vi "fullSERVER - SegnNotDAQ.vi"() -> ()   [LabVIEW 2023]
uses:
  <vilib>/Waveform/WDTFileIO.llb/Read Waveform from File.vi
panel:
  in  "file path (dialog if empty)":path
  out "SIGNAL":waveform(dbl)(graph)
  out "# POINTS":dbl
  out "OBSERVATION TIME":dbl
  out "SAMPLING FREQUENCY":dbl
  in  "PORT":u16
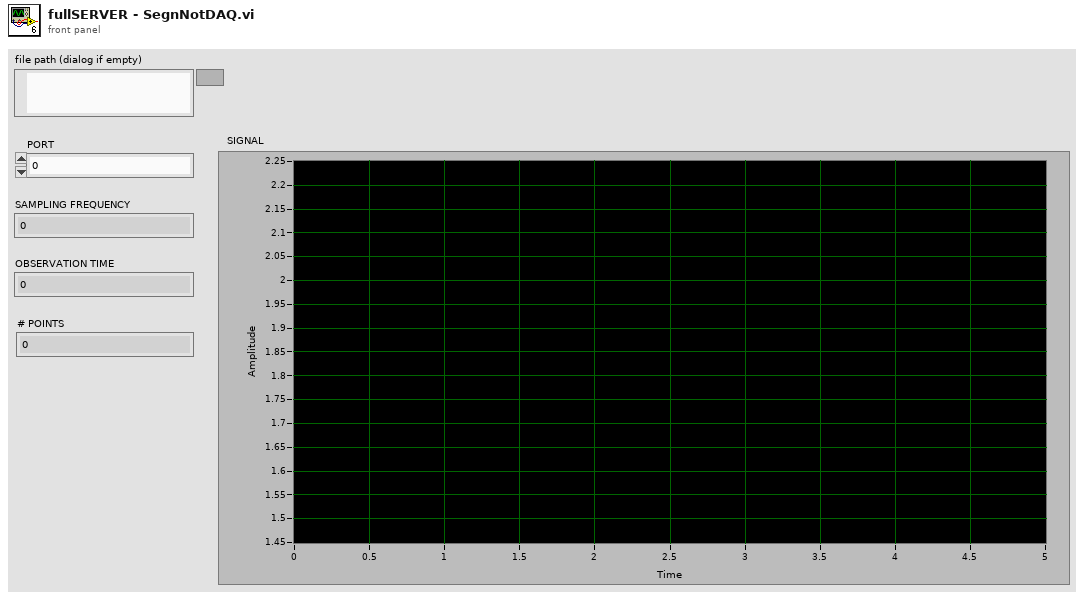
[diagram p1: front panel]
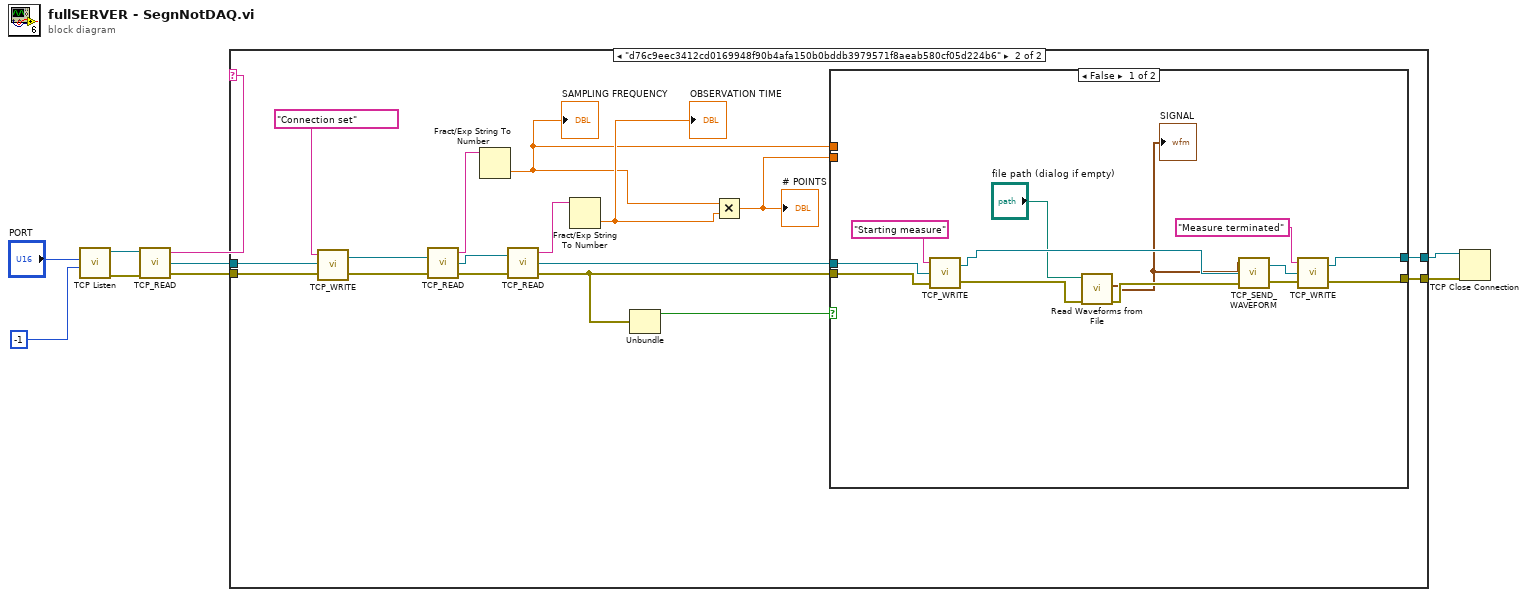
[diagram p0: block diagram]
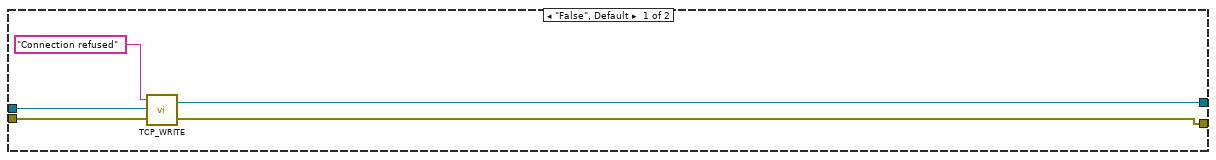
[diagram p2: hidden frame]
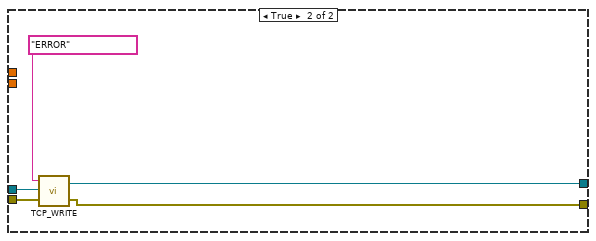
[diagram p3: hidden frame]
diagram:
  n1 = call <vilib>:"TCP Listen.vi"("timeout ms (wait forever: -1)"=-1, "port"="PORT") -> ("error out"=w6:errorcluster, "connection ID"=w7:refnum<k5>)  [unwired: 5 in, 3 out]
  n2 = call "TCP_READ.vi"("connection ID"=w7, "error in (no error)"=w6) -> ("data"=w5:string, "connection ID out"=w4:refnum<k5>, "error out"=w3:errorcluster)
  n3 = case shown="\"d76c9eec3412cd0169948f90b4afa150b0bddb3979571f8aeab580cf05d224b6\"" w5 {
    tunnel: w4 -> [w13 w30]
    tunnel: w3 -> [w14 w31]
    tunnel: [w12 w17] -> w2
    tunnel: [w11 w18] -> w1
    frame "False", Default {
      n4 = call "TCP_WRITE.vi"("error in (no error)"=w14, "connection ID"=w13, "data"="Connection refused") -> ("error out"=w11:errorcluster, "connection ID out"=w12:refnum<k5>)
    }
    frame "d76c9eec3412cd0169948f90b4afa150b0bddb3979571f8aeab580cf05d224b6" {
      n5 = call "TCP_WRITE.vi"("error in (no error)"=w31, "connection ID"=w30, "data"="Connection set") -> ("error out"=w28:errorcluster, "connection ID out"=w27:refnum<k5>)
      n6 = call "TCP_READ.vi"("connection ID"=w27, "error in (no error)"=w28) -> ("data"=w24:string, "connection ID out"=w25:refnum<k5>, "error out"=w26:errorcluster)
      n7 = Fract/Exp String To Number(string=w24) -> (number=w16:dbl)  [unwired: 3 in, 1 out]
      "SAMPLING FREQUENCY" <- w16
      n8 = call "TCP_READ.vi"("connection ID"=w25, "error in (no error)"=w26) -> ("data"=w23:string, "connection ID out"=w21:refnum<k5>, "error out"=w20:errorcluster)
      n9 = Fract/Exp String To Number(string=w23) -> (number=w22:dbl)  [unwired: 3 in, 1 out]
      "OBSERVATION TIME" <- w22
      n10 = Unbundle(w20) -> ("status"=w19:bool)  [unwired: 2 out]
      n11 = Multiply(x=w16, y=w22) -> (x*y=w15:dbl)
      "# POINTS" <- w15
      n12 = case shown="False" w19 {
        tunnel: w20 -> [w44 w49]
        tunnel: w21 -> [w43 w48]
        tunnel: [w38 w46] -> w17
        tunnel: [w37 w45] -> w18
        tunnel: w16 -> [_ _]
        tunnel: w15 -> [_ _]
        frame False {
          n13 = call "TCP_WRITE.vi"("error in (no error)"=w44, "connection ID"=w43, "data"="Starting measure") -> ("error out"=w35:errorcluster, "connection ID out"=w41:refnum<k5>)
          n14 = call-poly <vilib>:"Read Waveforms from File.vi"("error in (no error)"=w35, "file path (dialog if empty)"="file path (dialog if empty)") -> ("error out"=w34:errorcluster, "first waveform in record"=w32:waveform(dbl))  [unwired: 4 in, 2 out]
          "SIGNAL" <- w32
          n15 = call "TCP_SEND_WAVEFORM.vi"("error in (no error)"=w34, "connection ID"=w41, "waveform"=w32) -> ("error out"=w40:errorcluster, "connection ID out"=w39:refnum<k5>)
          n16 = call "TCP_WRITE.vi"("error in (no error)"=w40, "connection ID"=w39, "data"="Measure terminated") -> ("error out"=w37:errorcluster, "connection ID out"=w38:refnum<k5>)
        }
        frame True {
          n17 = call "TCP_WRITE.vi"("error in (no error)"=w49, "connection ID"=w48, "data"="ERROR") -> ("error out"=w45:errorcluster, "connection ID out"=w46:refnum<k5>)
        }
      }
    }
  }
  n18 = TCP Close Connection(connection ID=w2, error in (no error)=w1) -> ()  [unwired: 1 in, 2 out]
